vi "执行下子.vi"(0 "当前棋盘状态":i32[][](array[numeric]), 7 "行":sgl, 9 "列":i16, 11 "白子/黑子?":i32) -> (3 "控制数组":bool[][](array[boolean]), 4 "当前棋盘状态":i32[][](array[numeric]), 8 "行":sgl, 10 "列":i16)   [LabVIEW 2018]
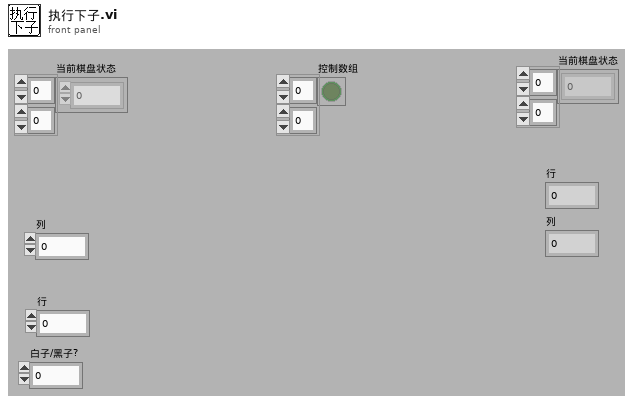
[diagram p1: front panel]
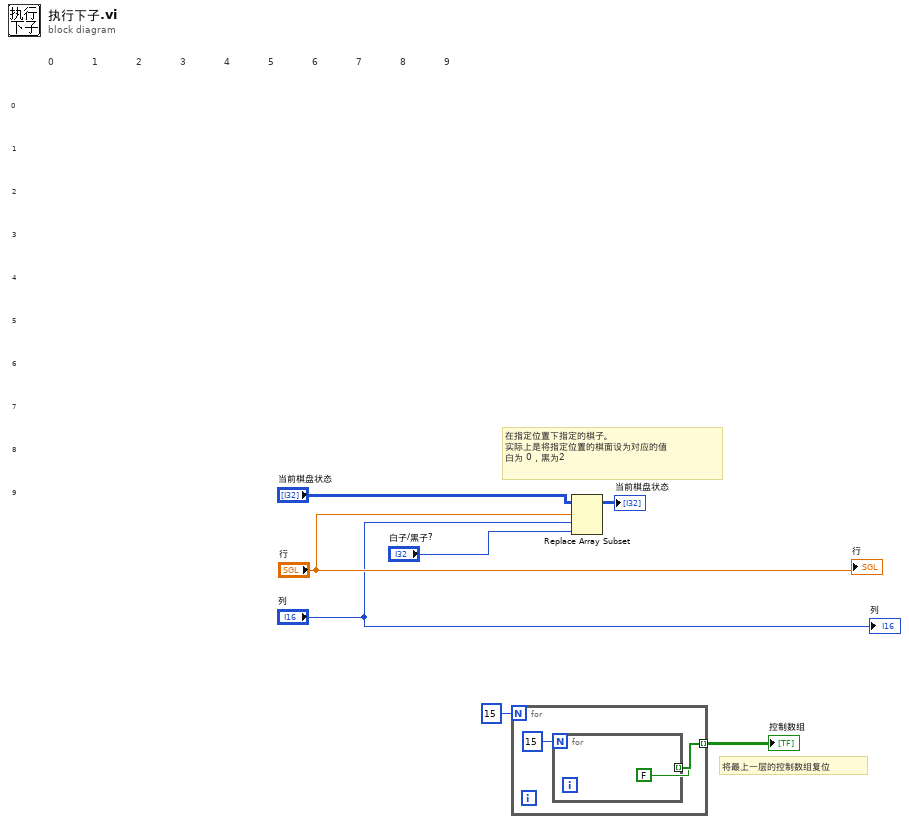
[diagram p0: block diagram]
diagram:
  # "在指定位置下指定的棋子。\n实际上是将指定位置的棋面设为对应的值\n白为 0，黑为2"
  # "将最上一层的控制数组复位"
  # "9"
  # "8"
  # "7"
  # "6"
  # "5"
  # "4"
  # "3"
  # "2"
  # "1"
  # "0"
  # "9"
  # "8"
  # "7"
  # "6"
  # "5"
  # "4"
  # "3"
  # "2"
  # "1"
  # "0"
  n1 = for {
    N: 15 -> [_]
    tunnel: [w9] -> w2 mode=indexing
    n2 = for {
      N: 15 -> [_]
      tunnel: [FALSE] -> w9 mode=indexing
    }
  }
  "控制数组" <- w2
  n3 = Replace Array Subset(array="当前棋盘状态", new element="白子/黑子?", index (row)="行", index (col)="列") -> (→"当前棋盘状态":i32[][])
  "行" <- "行"
  "列" <- "列"
